vi "Больше И.vi"(1 "Чек":bool, 2 "Граница":dbl, 3 "Значение":dbl) -> (0 "T/F":bool)   [LabVIEW 2018]
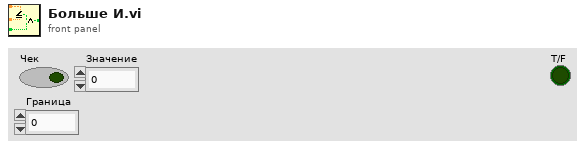
[diagram p1: front panel]
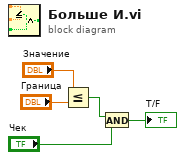
[diagram p0: block diagram]
diagram:
  n1 = Less Or Equal?(x="Значение", y="Граница") -> (x <= y?=w5:bool)
  n2 = And(x=w5, y="Чек") -> (x .and. y?=→"T/F":bool)
